vi "Mode_Write.vi"(4 "error in (no error)":errorcluster, 5 "Value":u8, 6 "Container State":T2, 7 "Display State In":T1 {"Mode" items=["U DC", "U AC", "I DC", "I AC", "R"]}) -> (0 "error out":errorcluster, 3 "Display State Out":T1 {"Mode" items=["U DC", "U AC", "I DC", "I AC", "R"]})   [LabVIEW 2020, in "Multimetr.xctl"]
uses:
  Multimetr.xctl
  <vilib>/_xctls/Container State.ctl
  Multimetr-state.ctl
  <vilib>/_xctls/XControlSupport.lvlib
panel:
  # "Replace the Value Control below with a Control of desired type.\nDo not remove this Control or the others from the connector pane.\nDo not change the connector pane pattern.\nThe Value control should always be the third terminal from top on the input side in the connector pane."
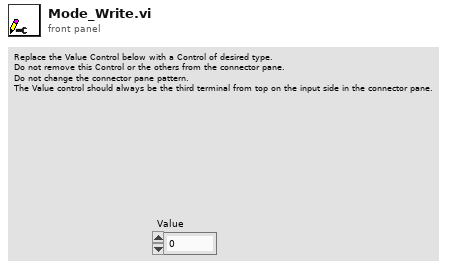
[diagram p1: front panel]
types:
  T1 = typedef "Multimetr.xctl/Multimetr-state.ctl" = cluster{"ON":bool, "Mode":u16, "I connected?":bool, "U connected?":bool}
  T2 = typedef "XControlSupport.lvlib/Container State.ctl" = cluster{"Indicator?":bool, "Run Mode?":bool, " Refnum":refnum<vi>}
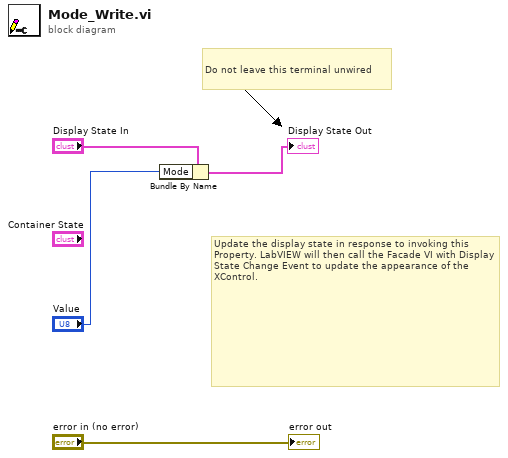
[diagram p0: block diagram]
diagram:
  # "Do not leave this terminal unwired"
  # "Update the display state in response to invoking this Property. LabVIEW will then call the Facade VI with Display State Change Event to update the appearance of the XControl."
  n1 = Bundle By Name(cluster="Display State In", "Mode"="Value") -> (→"Display State Out":T1)
  "error out" <- "error in (no error)"
